vi "Revision Query.vi"(0 "VISA resource name":refnum<visa-resource-name>, 11 "error in (no error)":errorcluster) -> (4 "VISA resource name out":refnum<visa-resource-name>, 6 "Instrument Driver Revision":string, 8 "Instrument Firmware Revision":string, 10 "Instrument Model":string, 15 "error out":errorcluster)   [LabVIEW 2016, in "APT 300XAC Series.lvlib"]
doc: "Queries the current instrument firmware revision and instrument driver revision.\n\nRefer to the Readme file for detailed driver information including modification history."
uses:
  APT 300XAC Series.lvlib
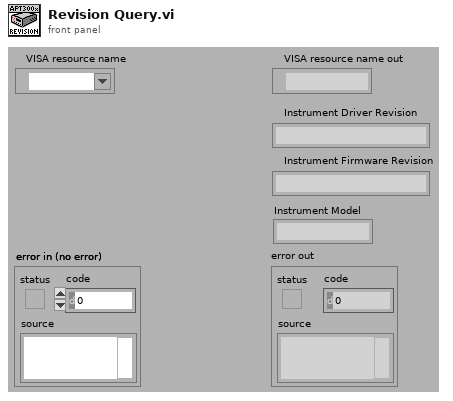
[diagram p1: front panel]
types:
  T1 = enum32{"invalid app kind", "Development System", "Run Time System", "Student Edition", "Embedded LabVIEW", "Evaluation", "Custom"}
  T2 = cluster{"Major":u16, "Minor":u16, "Fix":u16, "Build":u16}
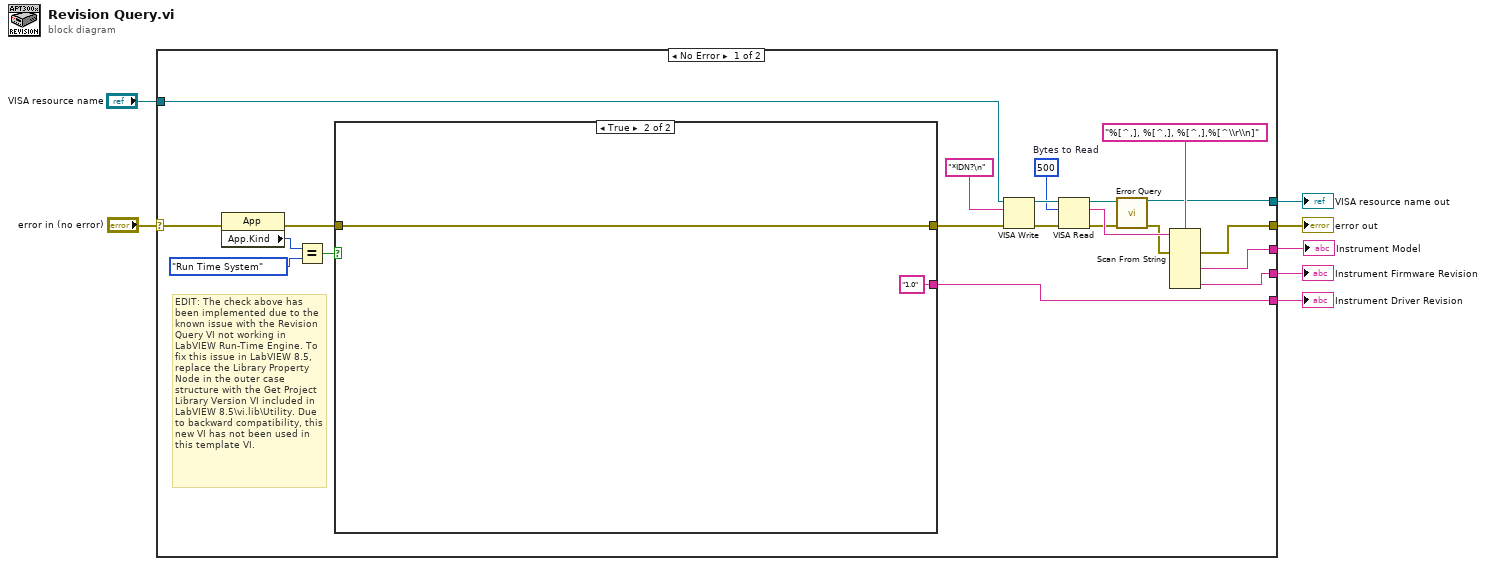
[diagram p0: block diagram]
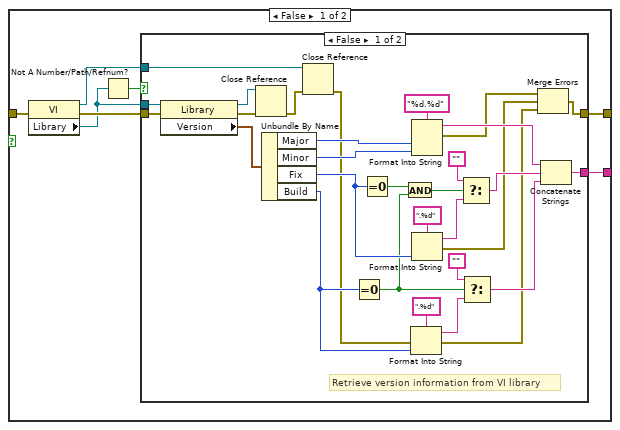
[diagram p2: hidden frame]
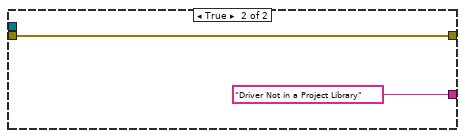
[diagram p3: hidden frame]
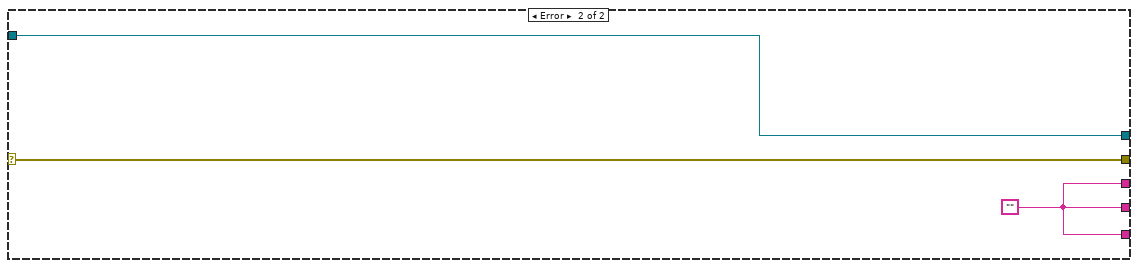
[diagram p4: hidden frame]
diagram:
  n1 = case shown="No Error" "error in (no error)" {
    selector: "error in (no error)" -> [w17 w72]
    tunnel: "VISA resource name" -> [w28 w71]
    tunnel: [w15 w70] -> w2
    tunnel: [w11 w71] -> w6
    tunnel: [w8 w72] -> w1
    tunnel: [w16 w70] -> w5
    tunnel: [w13 w70] -> w3
    frame No Error {
      w18 = u32 500  # Bytes to Read
      # "EDIT: The check above has been implemented due to the known issue with the Revision Query VI not working in LabVIEW Run-Time Engine. To fix this issue in LabVIEW 8.5, replace the Library Property Node in the outer case structure with the Get Project Library Version VI included in LabVIEW 8.5\\vi.lib\\Utility. Due to backward compatibility, this new VI has not been used in this template VI."
      n2 = property on="Property Node" class="App"(error in=w17) -> (error out=w19:errorcluster, "App.Kind"=w21:T1)  [unwired: 1 in, 1 out]
      n3 = Equal?(x=w21, y=T1."Run Time System" ("Application:Kind")) -> (x = y?=w22:bool)
      n4 = case shown="True" w22 {
        tunnel: [w31 "1.0"] -> w16
        tunnel: w19 -> [w30 w68]
        tunnel: [w29 w68] -> w23
        frame False {
          n5 = property on="Property Node" class="VI"(error in=w30) -> (reference out=w35:refnum<vi>, error out=w34:errorcluster, "Library"=w33:refnum<vi>)  [unwired: 1 in]
          n6 = Not A Number/Path/Refnum?(number/path/refnum=w33) -> (NaN/Path/Refnum?=w32:bool)
          n7 = case shown="False" w32 {
            tunnel: w35 -> [w62 _]
            tunnel: w34 -> [w47 w67]
            tunnel: [w36 w67] -> w29
            tunnel: [w42 "Driver Not in a Project Library"] -> w31
            tunnel: w33 -> [w41 _]
            frame False {
              # "Retrieve version information from VI library"
              n8 = property on="Property Node" class="Library"(reference=w41, error in=w47) -> (reference out=w64:refnum<vi>, error out=w65:errorcluster, "Version"=w61:T2)
              n9 = Close Reference(reference=w64, error in (no error)=w65) -> (error out=w63:errorcluster)
              n10 = Unbundle By Name(w61) -> ("Major"=w50:u16, "Minor"=w49:u16, "Fix"=w46:u16, "Build"=w48:u16)
              n11 = Close Reference(reference=w62, error in (no error)=w63) -> (error out=w40:errorcluster)
              n12 = Equal To 0?(x=w48) -> (x = 0?=w44:bool)
              n13 = Equal To 0?(x=w46) -> (x = 0?=w45:bool)
              n14 = And(x=w45, y=w44) -> (x .and. y?=w43:bool)
              n15 = Format Into String(format string=".%d", error in=w40, w48) -> (resulting string=w54:string, error out=w37:errorcluster)  [unwired: 1 in]
              n16 = Format Into String(format string="%d.%d", w50, w49) -> (resulting string=w56:string, error out=w39:errorcluster)  [unwired: 2 in]
              n17 = Format Into String(format string=".%d", w46) -> (resulting string=w58:string, error out=w38:errorcluster)  [unwired: 2 in]
              n18 = Select(t="" ("Empty String Constant"), s=w43, f=w58) -> (s? t:f=w55:string)
              n19 = Select(t="" ("Empty String Constant"), s=w44, f=w54) -> (s? t:f=w51:string)
              n20 = Merge Errors(w39, w38, w37) -> (w36:errorcluster)
              n21 = Concatenate Strings(w56, w55, w51) -> (w42:string)
            }
            frame True {
            }
          }
        }
        frame True {
        }
      }
      n22 = VISA Write(VISA resource name=w28, write buffer="*IDN?\n", error in (no error)=w23) -> (VISA resource name out=w27:refnum<visa-resource-name>, error out=w26:errorcluster)  [unwired: 1 out]
      n23 = VISA Read(VISA resource name=w27, byte count=w18, error in (no error)=w26) -> (VISA resource name out=w12:refnum<visa-resource-name>, read buffer=w14:string, error out=w10:errorcluster)  [unwired: 1 out]
      n24 = call "Error Query.vi"("VISA resource name"=w12, "error in (no error)"=w10) -> ("VISA resource name out"=w11:refnum<visa-resource-name>, "error out"=w9:errorcluster)  [unwired: 10 in, 2 out]
      n25 = Scan From String(format string="%[^,], %[^,], %[^,],%[^\\r\\n]", input string=w14, error in=w9) -> (error out=w8:errorcluster, output 2=w13:string, output 4=w15:string)  [unwired: 7 in, 2 out]
    }
    frame Error {
      w70 = "" ("Empty String Constant")
    }
  }
  "Instrument Firmware Revision" <- w2
  "Instrument Driver Revision" <- w5
  "VISA resource name out" <- w6
  "error out" <- w1
  "Instrument Model" <- w3
